vi "Put-Ball-Lite_Test.vi"() -> ()   [LabVIEW 2019]
uses:
  <vilib>/myRIO/Common/Instrument Driver Framework/myRIO v1.0/UART/vis/myRIO v1.0 Close UART.vi
  <vilib>/myRIO/Common/Instrument Driver Framework/Utilities/vis/FPGA Ref Manager.vi
  <vilib>/myRIO/Common/Instrument Driver Framework/myRIO v1.0/myRIO v1.0 Reset FPGA.vi
  <vilib>/myRIO/Common/Instrument Driver Framework/myRIO v1.0/IRQ/vis/myRIO v1.0 IRQ Info FGV.vi
  <vilib>/myRIO/Common/Instrument Driver Framework/myRIO v1.0/IRQ/vis/myRIO v1.0 Timer IRQ Info FGV.vi
  <vilib>/myRIO/Common/Instrument Driver Framework/myRIO v1.0/IRQ/vis/myRIO v1.0 ISR Agent.vi
  <vilib>/myRIO/Instrument Drivers/Utilities/vis/Reset Index.vi
  <vilib>/myRIO/Common/Instrument Driver Framework/myRIO v1.0/Resource Manager/vis/myRIO v1.0 Block Write Resource Manager.vi
  <vilib>/myRIO/Instrument Drivers/Utilities/Utilities.lvlib
panel:
  out "Error Out":errorcluster
  in  "Stop":bool
  out "輸出顏色-位置 2":T1(array[cluster])
  in  "Error In":errorcluster
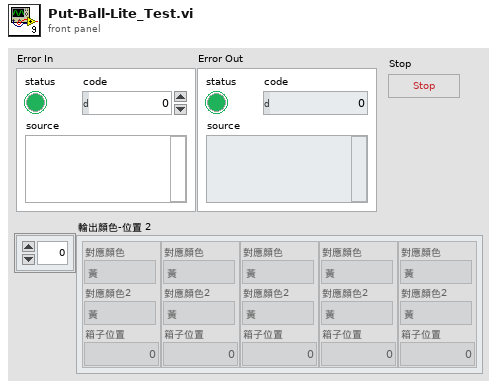
[diagram p1: front panel]
types:
  T1 = cluster{"對應顏色":enum16{"黃", "紅", "綠", "藍", "黑", "無"}, "對應顏色2":enum16{"黃", "紅", "綠", "藍", "黑", "無"}, "箱子位置":i32}[]
  T2 = typedef "I2C.lvlib/I2C Reference.ctl" = cluster{"myRIO Reference":T3, "I2C Channels Enum":T7, "I2C Configuration":T8}
  T3 = typedef "myRIO Generic Hardware Reference.ctl" = cluster{"myRIO Model":T4, "myRIO Hardware Reference":T5}
  T4 = typedef "Hardware Version Enum.ctl" = enum16{"Unknown", "myRIO-1900", "myRIO-1950", "roboRIO", "NI ELVIS RIO CM", "ELVIS III"}
  T5 = typedef "myRIO v1.0 Reference.ctl" = cluster{"Generic FPGA Reference":T6, "Allow multiple opens":bool}
  T6 = typedef "Generic FPGA Reference.ctl" = refnum<k20>
  T7 = typedef "I2C Channels Enum.ctl" = enum16{"Not Connected", "A/I2C", "B/I2C", "I2C/I2C"}
  T8 = typedef "I2C.lvlib/I2C Configuration.ctl" = cluster{"I2C Transfer Rate":T9}
  T9 = typedef "I2C.lvlib/I2C Transfer Rate.ctl" = enum16{"Standard mode (100 kbps)", "Fast mode (400 kbps)"}
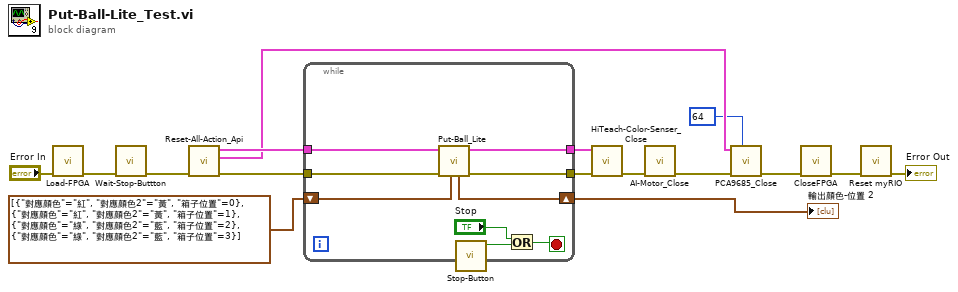
[diagram p0: block diagram]
diagram:
  n1 = call "Load-FPGA.vi"("Error In"="Error In") -> ("Error Out"=w15:errorcluster)  [unwired: 10 in]
  n2 = call "Wait-Stop-Buttton.vi"("Error In"=w15) -> ("Error Out"=w16:errorcluster)  [unwired: 10 in]
  n3 = call "Reset-All-Action_Api.vi"("Error In"=w16) -> ("Error Out"=w13:errorcluster, "I2C Ref Out"=w3:T2, "HiTechnicColorSensorV2 Ref Out"=w11:cluster{"I2C Ref Out":T2})  [unwired: 8 in]
  n4 = while {
    tunnel: w13 -> [w22]
    tunnel: w11 -> [w21]
    shift-right: [w18] -> w10
    shift-left: T1 [{"對應顏色"=enum."紅", "對應顏色2"=enum."黃", "箱子位置"=0}, {"對應顏色"=enum."紅", "對應顏色2"=enum."黃", "箱子位置"=1}, {"對應顏色"=enum."綠", "對應顏色2"=enum."藍", "箱子位置"=2}, {"對應顏色"=enum."綠", "對應顏色2"=enum."藍", "箱子位置"=3}] ("輸出顏色-位置") -> [w17]
    tunnel: [w20] -> w8
    tunnel: [w19] -> w7
    stop <- w25 stop-if-true
    n5 = call "Put-Ball_Lite.vi"("輸出顏色-位置"=w17, "Error In"=w22, "HiTechnicColorSensorV2 Ref In"=w21) -> ("Error Out"=w19:errorcluster, "HiTechnicColorSensorV2 Ref Out"=w20:cluster{"I2C Ref Out":T2}, "輸出顏色-位置"=w18:T1)  [unwired: 6 in]
    n6 = call "Stop-Button.vi"() -> ("顯示按下?"=w24:bool)  [unwired: 10 in, 1 out]
    n7 = Or(x="Stop", y=w24) -> (x .or. y?=w25:bool)
  }
  "輸出顏色-位置 2" <- w10
  n8 = call "HiTeach-Color-Senser_Close.vi"("Error In"=w7, "HiTechnicColorSensorV2 Ref"=w8) -> ("Error Out"=w4:errorcluster)  [unwired: 9 in]
  n9 = call "AI-Motor_Close.vi"("Error In"=w4) -> ("Error Out"=w2:errorcluster)  [unwired: 10 in]
  n10 = call "PCA9685_Close.vi"("驅動板位址(0x40)"=u8 64, "Error In"=w2, "I2C Ref In"=w3) -> ("Error Out"=w5:errorcluster)  [unwired: 8 in]
  n11 = call "CloseFPGA.vi"("Error In"=w5) -> ("Error Out"=w12:errorcluster)  [unwired: 10 in]
  n12 = call <vilib>:"Reset myRIO.vi"("error in (no error)"=w12) -> ("error out"=→"Error Out":errorcluster)  [unwired: 10 in]
